vi "Live.GetChannelInfo.vi"(8 "error in (no error)":errorcluster, 10 "Item URL":string, 11 "OPC UA client refnum in":refnum<k21>) -> (0 "error out":errorcluster, 1 "Setings":T1={"Settings"={"name"="", "node type"=enum."Other", "DataType"=1, "access"=enum."Null", "description"=""}, "Array Size"=0} {"Settings"."DataType" items=["Boolean"=1, "SByte"=2, "Byte"=3, "Int16"=4, "UInt16"=5, "Int32"=6, "UInt32"=7, "Int64"=8, "UInt64"=9, "Float"=10, "Double"=11, "String"=12, "DateTime"=13, "ByteString"=15, "Array of Boolean"=101, "Array of SByte"=102, "Array of Byte"=103, "Array of Int16"=104, "Array of UInt16"=105, "Array of Int32"=106, "Array of UInt32"=107, "Array of Int64"=108, "Array of UInt64"=109, "Array of Float"=110, "Array of Double"=111, "Array of String"=112, "Array of DateTime"=113, "Array of ByteString"=115]}, 2 "Item URL out":string, 3 "OPC UA client refnum out":refnum<k21>, 4 "Use":bool)   [LabVIEW 2013, in "OPC UA Client System Explorer.lvlib"]
uses:
  OPC UA Client System Explorer.lvlib
  Types/Tag.Settings
  <vilib>/OPCUA/client/Read ByteString.vi
  <vilib>/OPCUA/client/Read Double Array.vi
  <vilib>/OPCUA/client/Read Float Array.vi
  <vilib>/OPCUA/client/Read UInt32 Array.vi
  <vilib>/OPCUA/client/Read Int32 Array.vi
  <vilib>/OPCUA/client/Read UInt16 Array.vi
  <vilib>/OPCUA/client/Read Int16 Array.vi
  <vilib>/OPCUA/client/Read Byte Array.vi
  <vilib>/OPCUA/client/Read SByte Array.vi
  <vilib>/OPCUA/client/Read Bool Array.vi
  <vilib>/OPCUA/client/Read UInt64 Array.vi
  <vilib>/OPCUA/client/Read Int64 Array.vi
  <vilib>/OPCUA/client/Read DateTime Array.vi
  Engine/OPC UA Client Engine.lvlib
  <vilib>/OPCUA/NI OPC UA Client.lvlib
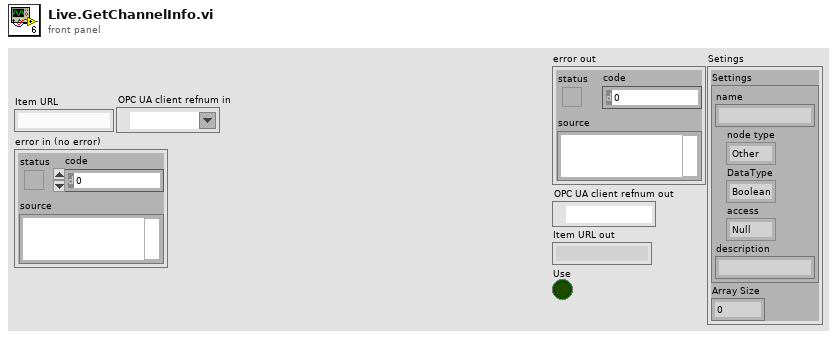
[diagram p1: front panel]
types:
  T1 = typedef "OPC UA Client Engine.lvlib/Tag.Settings" = cluster{"Settings":cluster{"name":string, "node type":enum32{"Other", "Folder", "Item/Property"}, "DataType":u32, "access":enum16{"Null", "Read", "Write", "Read&Write"}, "description":string}, "Array Size":i32}
  T2 = cluster{"name":string, "node type":enum32{"Other", "Folder", "Item/Property"}, "DataType":u32, "access":enum16{"Null", "Read", "Write", "Read&Write"}, "description":string}
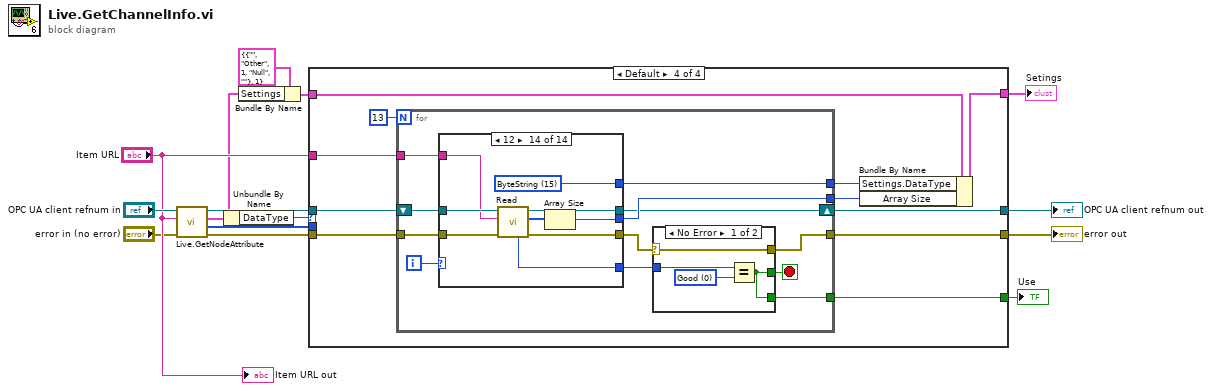
[diagram p0: block diagram]
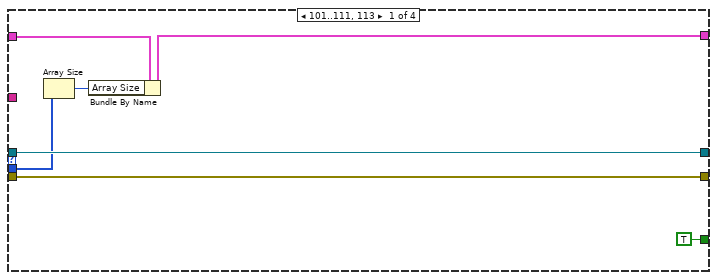
[diagram p2: hidden frame]
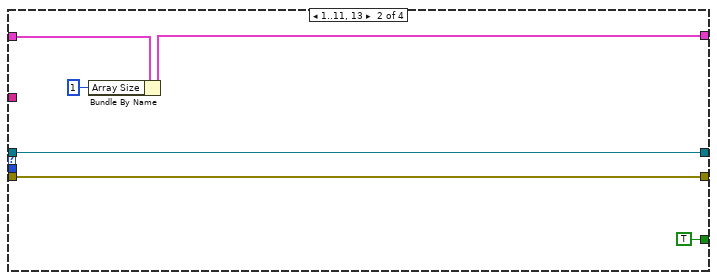
[diagram p3: hidden frame]
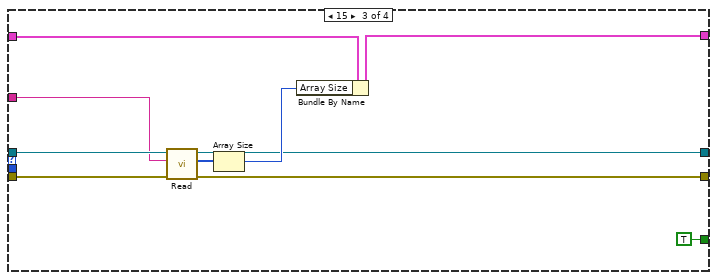
[diagram p4: hidden frame]
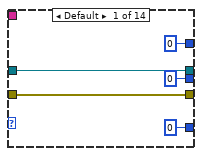
[diagram p5: hidden frame]
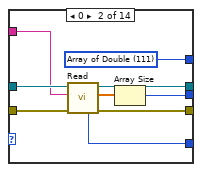
[diagram p6: hidden frame]
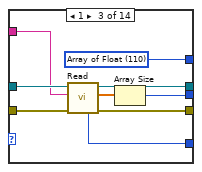
[diagram p7: hidden frame]
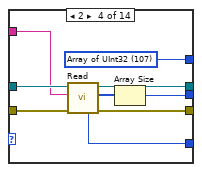
[diagram p8: hidden frame]
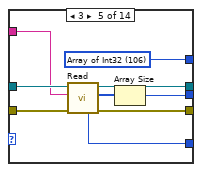
[diagram p9: hidden frame]
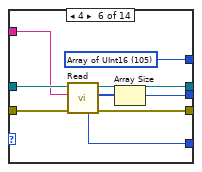
[diagram p10: hidden frame]
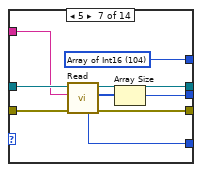
[diagram p11: hidden frame]
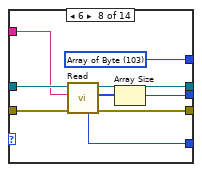
[diagram p12: hidden frame]
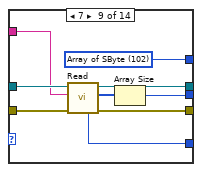
[diagram p13: hidden frame]
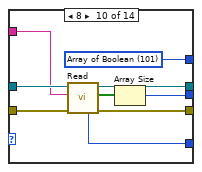
[diagram p14: hidden frame]
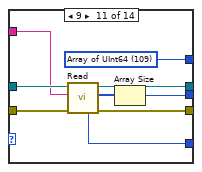
[diagram p15: hidden frame]
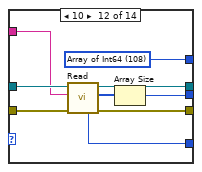
[diagram p16: hidden frame]
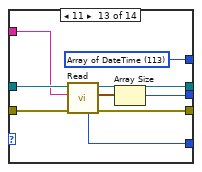
[diagram p17: hidden frame]
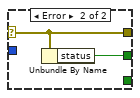
[diagram p18: hidden frame]
diagram:
  n1 = call "Live.GetNodeAttribute.vi"("error in (no error)"="error in (no error)", "node path"="Item URL", "OPC UA client refnum in"="OPC UA client refnum in") -> ("error out"=w6:errorcluster, "status"=w3:u32[], "node attribute"=w4:T2, "OPC UA client refnum out"=w5:refnum<k21>)  [unwired: 5 in]
  n2 = Unbundle By Name(w4) -> ("DataType"=w11:u32)
  n3 = Bundle By Name(cluster=T1 {"Settings"={"name"="", "node type"=enum."Other", "DataType"=1, "access"=enum."Null", "description"=""}, "Array Size"=1}, "Settings"=w4) -> (w10:T1)
  n4 = case shown="Default" w11 {
    tunnel: [w18 w24 w28 w40] -> w14
    tunnel: [w19 w25 w29 w39] -> w13
    tunnel: w6 -> [w18 w24 w33 w45]
    tunnel: w5 -> [w19 w25 w32 w43]
    tunnel: "Item URL" -> [_ _ w31 w44]
    tunnel: w10 -> [w21 w27 w37 w48]
    tunnel: [w20 w26 w36 w47] -> w2
    tunnel: w3 -> [w17 _ _ _]
    tunnel: [TRUE ("status") TRUE ("status") TRUE ("status") w38] -> w1
    frame 101..111, 113 {
      n5 = Array Size(array=w17) -> (size(s)=w16:i32)
      n6 = Bundle By Name(cluster=w21, "Array Size"=w16) -> (w20:T1)
    }
    frame 1..11, 13 {
      n7 = Bundle By Name(cluster=w27, "Array Size"=1) -> (w26:T1)
    }
    frame 15 {
      n8 = call-poly <vilib>:"Read.vi"("error in (no error)"=w33, "node path"=w31, "OPC UA client refnum in"=w32) -> ("error out"=w28:errorcluster, "value"=w34:u8[], "OPC UA client refnum out"=w29:refnum<k21>)  [unwired: 4 in, 2 out]
      n9 = Array Size(array=w34) -> (size(s)=w30:i32)
      n10 = Bundle By Name(cluster=w37, "Array Size"=w30) -> (w36:T1)
    }
    frame Default {
      n11 = for {
        N: 13 -> [_]
        tunnel: w45 -> [w60]
        tunnel: w44 -> [w58]
        tunnel: [w55] -> w40
        tunnel: [w53] -> w41
        tunnel: [w52] -> w42
        shift-right: [w51] -> w39
        shift-left: w43 -> [w59]
        tunnel: [w49] -> w38
        i -> [w54]
        stop <- w50 stop-if-true
        n12 = case shown="12" w54 {
          tunnel: w60 -> [w63 w74 w83 w92 w101 w110 w119 w128 w137 w146 w155 w164 w173 w182]
          tunnel: w59 -> [w61 w73 w82 w91 w100 w109 w118 w127 w136 w145 w154 w163 w172 w181]
          tunnel: w58 -> [_ w72 w81 w90 w99 w108 w117 w126 w135 w144 w153 w162 w171 w180]
          tunnel: [w63 w71 w80 w89 w98 w107 w116 w125 w134 w143 w152 w161 w170 w179] -> w57
          tunnel: [u32 0 ("status") w70 w79 w88 w97 w106 w115 w124 w133 w142 w151 w160 w169 w178] -> w56
          tunnel: [u32 0 ("DataType") w68 w77 w86 w95 w104 w113 w122 w131 w140 w149 w158 w167 w176] -> w52
          tunnel: [0 w67 w76 w85 w94 w103 w112 w121 w130 w139 w148 w157 w166 w175] -> w53
          tunnel: [w61 w66 w75 w84 w93 w102 w111 w120 w129 w138 w147 w156 w165 w174] -> w51
          frame Default {
          }
          frame 0 {
            w68 = u32 111 items=["Boolean"=1, "SByte"=2, "Byte"=3, "Int16"=4, "UInt16"=5, "Int32"=6, "UInt32"=7, "Int64"=8, "UInt64"=9, "Float"=10, "Double"=11, "String"=12, "DateTime"=13, "ByteString"=15, "Array of Boolean"=101, "Array of SByte"=102, "Array of Byte"=103, "Array of Int16"=104, "Array of UInt16"=105, "Array of Int32"=106, "Array of UInt32"=107, "Array of Int64"=108, "Array of UInt64"=109, "Array of Float"=110, "Array of Double"=111, "Array of String"=112, "Array of DateTime"=113, "Array of ByteString"=115] ("DataType")
            n13 = call-poly <vilib>:"Read.vi"("error in (no error)"=w74, "node path"=w72, "OPC UA client refnum in"=w73) -> ("error out"=w71:errorcluster, "value"=w69:dbl[], "OPC UA client refnum out"=w66:refnum<k21>, "status"=w70:u32)  [unwired: 4 in, 1 out]
            n14 = Array Size(array=w69) -> (size(s)=w67:i32)
          }
          frame 1 {
            w77 = u32 110 items=["Boolean"=1, "SByte"=2, "Byte"=3, "Int16"=4, "UInt16"=5, "Int32"=6, "UInt32"=7, "Int64"=8, "UInt64"=9, "Float"=10, "Double"=11, "String"=12, "DateTime"=13, "ByteString"=15, "Array of Boolean"=101, "Array of SByte"=102, "Array of Byte"=103, "Array of Int16"=104, "Array of UInt16"=105, "Array of Int32"=106, "Array of UInt32"=107, "Array of Int64"=108, "Array of UInt64"=109, "Array of Float"=110, "Array of Double"=111, "Array of String"=112, "Array of DateTime"=113, "Array of ByteString"=115] ("DataType")
            n15 = call-poly <vilib>:"Read.vi"("error in (no error)"=w83, "node path"=w81, "OPC UA client refnum in"=w82) -> ("error out"=w80:errorcluster, "value"=w78:sgl[], "OPC UA client refnum out"=w75:refnum<k21>, "status"=w79:u32)  [unwired: 4 in, 1 out]
            n16 = Array Size(array=w78) -> (size(s)=w76:i32)
          }
          frame 2 {
            w86 = u32 107 items=["Boolean"=1, "SByte"=2, "Byte"=3, "Int16"=4, "UInt16"=5, "Int32"=6, "UInt32"=7, "Int64"=8, "UInt64"=9, "Float"=10, "Double"=11, "String"=12, "DateTime"=13, "ByteString"=15, "Array of Boolean"=101, "Array of SByte"=102, "Array of Byte"=103, "Array of Int16"=104, "Array of UInt16"=105, "Array of Int32"=106, "Array of UInt32"=107, "Array of Int64"=108, "Array of UInt64"=109, "Array of Float"=110, "Array of Double"=111, "Array of String"=112, "Array of DateTime"=113, "Array of ByteString"=115] ("DataType")
            n17 = call-poly <vilib>:"Read.vi"("error in (no error)"=w92, "node path"=w90, "OPC UA client refnum in"=w91) -> ("error out"=w89:errorcluster, "value"=w87:u32[], "OPC UA client refnum out"=w84:refnum<k21>, "status"=w88:u32)  [unwired: 4 in, 1 out]
            n18 = Array Size(array=w87) -> (size(s)=w85:i32)
          }
          frame 3 {
            w95 = u32 106 items=["Boolean"=1, "SByte"=2, "Byte"=3, "Int16"=4, "UInt16"=5, "Int32"=6, "UInt32"=7, "Int64"=8, "UInt64"=9, "Float"=10, "Double"=11, "String"=12, "DateTime"=13, "ByteString"=15, "Array of Boolean"=101, "Array of SByte"=102, "Array of Byte"=103, "Array of Int16"=104, "Array of UInt16"=105, "Array of Int32"=106, "Array of UInt32"=107, "Array of Int64"=108, "Array of UInt64"=109, "Array of Float"=110, "Array of Double"=111, "Array of String"=112, "Array of DateTime"=113, "Array of ByteString"=115] ("DataType")
            n19 = call-poly <vilib>:"Read.vi"("error in (no error)"=w101, "node path"=w99, "OPC UA client refnum in"=w100) -> ("error out"=w98:errorcluster, "value"=w96:i32[], "OPC UA client refnum out"=w93:refnum<k21>, "status"=w97:u32)  [unwired: 4 in, 1 out]
            n20 = Array Size(array=w96) -> (size(s)=w94:i32)
          }
          frame 4 {
            w104 = u32 105 items=["Boolean"=1, "SByte"=2, "Byte"=3, "Int16"=4, "UInt16"=5, "Int32"=6, "UInt32"=7, "Int64"=8, "UInt64"=9, "Float"=10, "Double"=11, "String"=12, "DateTime"=13, "ByteString"=15, "Array of Boolean"=101, "Array of SByte"=102, "Array of Byte"=103, "Array of Int16"=104, "Array of UInt16"=105, "Array of Int32"=106, "Array of UInt32"=107, "Array of Int64"=108, "Array of UInt64"=109, "Array of Float"=110, "Array of Double"=111, "Array of String"=112, "Array of DateTime"=113, "Array of ByteString"=115] ("DataType")
            n21 = call-poly <vilib>:"Read.vi"("error in (no error)"=w110, "node path"=w108, "OPC UA client refnum in"=w109) -> ("error out"=w107:errorcluster, "value"=w105:u16[], "OPC UA client refnum out"=w102:refnum<k21>, "status"=w106:u32)  [unwired: 4 in, 1 out]
            n22 = Array Size(array=w105) -> (size(s)=w103:i32)
          }
          frame 5 {
            w113 = u32 104 items=["Boolean"=1, "SByte"=2, "Byte"=3, "Int16"=4, "UInt16"=5, "Int32"=6, "UInt32"=7, "Int64"=8, "UInt64"=9, "Float"=10, "Double"=11, "String"=12, "DateTime"=13, "ByteString"=15, "Array of Boolean"=101, "Array of SByte"=102, "Array of Byte"=103, "Array of Int16"=104, "Array of UInt16"=105, "Array of Int32"=106, "Array of UInt32"=107, "Array of Int64"=108, "Array of UInt64"=109, "Array of Float"=110, "Array of Double"=111, "Array of String"=112, "Array of DateTime"=113, "Array of ByteString"=115] ("DataType")
            n23 = call-poly <vilib>:"Read.vi"("error in (no error)"=w119, "node path"=w117, "OPC UA client refnum in"=w118) -> ("error out"=w116:errorcluster, "value"=w114:i16[], "OPC UA client refnum out"=w111:refnum<k21>, "status"=w115:u32)  [unwired: 4 in, 1 out]
            n24 = Array Size(array=w114) -> (size(s)=w112:i32)
          }
          frame 6 {
            w122 = u32 103 items=["Boolean"=1, "SByte"=2, "Byte"=3, "Int16"=4, "UInt16"=5, "Int32"=6, "UInt32"=7, "Int64"=8, "UInt64"=9, "Float"=10, "Double"=11, "String"=12, "DateTime"=13, "ByteString"=15, "Array of Boolean"=101, "Array of SByte"=102, "Array of Byte"=103, "Array of Int16"=104, "Array of UInt16"=105, "Array of Int32"=106, "Array of UInt32"=107, "Array of Int64"=108, "Array of UInt64"=109, "Array of Float"=110, "Array of Double"=111, "Array of String"=112, "Array of DateTime"=113, "Array of ByteString"=115] ("DataType")
            n25 = call-poly <vilib>:"Read.vi"("error in (no error)"=w128, "node path"=w126, "OPC UA client refnum in"=w127) -> ("error out"=w125:errorcluster, "value"=w123:u8[], "OPC UA client refnum out"=w120:refnum<k21>, "status"=w124:u32)  [unwired: 4 in, 1 out]
            n26 = Array Size(array=w123) -> (size(s)=w121:i32)
          }
          frame 7 {
            w131 = u32 102 items=["Boolean"=1, "SByte"=2, "Byte"=3, "Int16"=4, "UInt16"=5, "Int32"=6, "UInt32"=7, "Int64"=8, "UInt64"=9, "Float"=10, "Double"=11, "String"=12, "DateTime"=13, "ByteString"=15, "Array of Boolean"=101, "Array of SByte"=102, "Array of Byte"=103, "Array of Int16"=104, "Array of UInt16"=105, "Array of Int32"=106, "Array of UInt32"=107, "Array of Int64"=108, "Array of UInt64"=109, "Array of Float"=110, "Array of Double"=111, "Array of String"=112, "Array of DateTime"=113, "Array of ByteString"=115] ("DataType")
            n27 = call-poly <vilib>:"Read.vi"("error in (no error)"=w137, "node path"=w135, "OPC UA client refnum in"=w136) -> ("error out"=w134:errorcluster, "value"=w132:i8[], "OPC UA client refnum out"=w129:refnum<k21>, "status"=w133:u32)  [unwired: 4 in, 1 out]
            n28 = Array Size(array=w132) -> (size(s)=w130:i32)
          }
          frame 8 {
            w140 = u32 101 items=["Boolean"=1, "SByte"=2, "Byte"=3, "Int16"=4, "UInt16"=5, "Int32"=6, "UInt32"=7, "Int64"=8, "UInt64"=9, "Float"=10, "Double"=11, "String"=12, "DateTime"=13, "ByteString"=15, "Array of Boolean"=101, "Array of SByte"=102, "Array of Byte"=103, "Array of Int16"=104, "Array of UInt16"=105, "Array of Int32"=106, "Array of UInt32"=107, "Array of Int64"=108, "Array of UInt64"=109, "Array of Float"=110, "Array of Double"=111, "Array of String"=112, "Array of DateTime"=113, "Array of ByteString"=115] ("DataType")
            n29 = call-poly <vilib>:"Read.vi"("error in (no error)"=w146, "node path"=w144, "OPC UA client refnum in"=w145) -> ("error out"=w143:errorcluster, "value"=w141:bool[], "OPC UA client refnum out"=w138:refnum<k21>, "status"=w142:u32)  [unwired: 4 in, 1 out]
            n30 = Array Size(array=w141) -> (size(s)=w139:i32)
          }
          frame 9 {
            w149 = u32 109 items=["Boolean"=1, "SByte"=2, "Byte"=3, "Int16"=4, "UInt16"=5, "Int32"=6, "UInt32"=7, "Int64"=8, "UInt64"=9, "Float"=10, "Double"=11, "String"=12, "DateTime"=13, "ByteString"=15, "Array of Boolean"=101, "Array of SByte"=102, "Array of Byte"=103, "Array of Int16"=104, "Array of UInt16"=105, "Array of Int32"=106, "Array of UInt32"=107, "Array of Int64"=108, "Array of UInt64"=109, "Array of Float"=110, "Array of Double"=111, "Array of String"=112, "Array of DateTime"=113, "Array of ByteString"=115] ("DataType")
            n31 = call-poly <vilib>:"Read.vi"("error in (no error)"=w155, "node path"=w153, "OPC UA client refnum in"=w154) -> ("error out"=w152:errorcluster, "value"=w150:u64[], "OPC UA client refnum out"=w147:refnum<k21>, "status"=w151:u32)  [unwired: 4 in, 1 out]
            n32 = Array Size(array=w150) -> (size(s)=w148:i32)
          }
          frame 10 {
            w158 = u32 108 items=["Boolean"=1, "SByte"=2, "Byte"=3, "Int16"=4, "UInt16"=5, "Int32"=6, "UInt32"=7, "Int64"=8, "UInt64"=9, "Float"=10, "Double"=11, "String"=12, "DateTime"=13, "ByteString"=15, "Array of Boolean"=101, "Array of SByte"=102, "Array of Byte"=103, "Array of Int16"=104, "Array of UInt16"=105, "Array of Int32"=106, "Array of UInt32"=107, "Array of Int64"=108, "Array of UInt64"=109, "Array of Float"=110, "Array of Double"=111, "Array of String"=112, "Array of DateTime"=113, "Array of ByteString"=115] ("DataType")
            n33 = call-poly <vilib>:"Read.vi"("error in (no error)"=w164, "node path"=w162, "OPC UA client refnum in"=w163) -> ("error out"=w161:errorcluster, "value"=w159:i64[], "OPC UA client refnum out"=w156:refnum<k21>, "status"=w160:u32)  [unwired: 4 in, 1 out]
            n34 = Array Size(array=w159) -> (size(s)=w157:i32)
          }
          frame 11 {
            w167 = u32 113 items=["Boolean"=1, "SByte"=2, "Byte"=3, "Int16"=4, "UInt16"=5, "Int32"=6, "UInt32"=7, "Int64"=8, "UInt64"=9, "Float"=10, "Double"=11, "String"=12, "DateTime"=13, "ByteString"=15, "Array of Boolean"=101, "Array of SByte"=102, "Array of Byte"=103, "Array of Int16"=104, "Array of UInt16"=105, "Array of Int32"=106, "Array of UInt32"=107, "Array of Int64"=108, "Array of UInt64"=109, "Array of Float"=110, "Array of Double"=111, "Array of String"=112, "Array of DateTime"=113, "Array of ByteString"=115] ("DataType")
            n35 = call-poly <vilib>:"Read.vi"("error in (no error)"=w173, "node path"=w171, "OPC UA client refnum in"=w172) -> ("error out"=w170:errorcluster, "value"=w168:timestamp[], "OPC UA client refnum out"=w165:refnum<k21>, "status"=w169:u32)  [unwired: 4 in, 1 out]
            n36 = Array Size(array=w168) -> (size(s)=w166:i32)
          }
          frame 12 {
            w176 = u32 15 items=["Boolean"=1, "SByte"=2, "Byte"=3, "Int16"=4, "UInt16"=5, "Int32"=6, "UInt32"=7, "Int64"=8, "UInt64"=9, "Float"=10, "Double"=11, "String"=12, "DateTime"=13, "ByteString"=15, "Array of Boolean"=101, "Array of SByte"=102, "Array of Byte"=103, "Array of Int16"=104, "Array of UInt16"=105, "Array of Int32"=106, "Array of UInt32"=107, "Array of Int64"=108, "Array of UInt64"=109, "Array of Float"=110, "Array of Double"=111, "Array of String"=112, "Array of DateTime"=113, "Array of ByteString"=115] ("DataType")
            n37 = call-poly <vilib>:"Read.vi"("error in (no error)"=w182, "node path"=w180, "OPC UA client refnum in"=w181) -> ("error out"=w179:errorcluster, "value"=w177:u8[], "OPC UA client refnum out"=w174:refnum<k21>, "status"=w178:u32)  [unwired: 4 in, 1 out]
            n38 = Array Size(array=w177) -> (size(s)=w175:i32)
          }
        }
        n39 = case shown="No Error" w57 {
          selector: w57 -> [w184 w187]
          tunnel: w56 -> [w186 _]
          tunnel: [w183 w188] -> w50
          tunnel: [w184 w187] -> w55
          tunnel: [w183 _] -> w49
          frame No Error {
            w185 = u32 0 items=["Good"=0, "Bad_AttributeIdInvalid"=2153906176, "Bad_BrowseDirectionInvalid"=2152529920, "Bad_BrowseNameInvalid"=2153775104, "Bad_ContentFilterInvalid"=2152202240, "Bad_ContinuationPointInvalid"=2152333312, "Bad_DataEncodingInvalid"=2151153664, "Bad_DataEncodingUnsupported"=2151219200, "Bad_EventFilterInvalid"=2152136704, "Bad_FilterNotAllowed"=2152005632, "Bad_FilterOperandInvalid"=2160132096, "Bad_HistoryOperationInvalid"=2154889216, "Bad_HistoryOperationUnsupported"=2154954752, "Bad_IndexRangeInvalid"=2151022592, "Bad_IndexRangeNoData"=2151088128, "Bad_MonitoredItemFilterInvalid"=2151874560, "Bad_MonitoredItemFilterUnsupported"=2151940096, "Bad_MonitoredItemIdInvalid"=2151809024, "Bad_MonitoringModeInvalid"=2151743488, "Bad_NoCommunication"=2150694912, "Bad_NoContinuationPoints"=2152398848, "Bad_NodeClassInvalid"=2153709568, "Bad_NodeIdInvalid"=2150825984, "Bad_NodeIdUnknown"=2150891520, "Bad_NoDeleteRights"=2154364928, "Bad_NodeNotInView"=2152595456, "Bad_NotFound"=2151546880, "Bad_NotImplemented"=2151677952, "Bad_NotReadable"=2151284736, "Bad_NotSupported"=2151481344, "Bad_NotWritable"=2151350272, "Bad_ObjectDeleted"=2151612416, "Bad_OutOfRange"=2151415808, "Bad_ReferenceTypeIdInvalid"=2152464384, "Bad_SourceNodeIdInvalid"=2154037248, "Bad_StructureMissing"=2152071168, "Bad_TargetNodeIdInvalid"=2154102784, "Bad_TypeDefinitionInvalid"=2153971712, "Bad_TypeMismatch"=2155085824, "Bad_WaitingForInitialData"=2150760448] ("status")
            n40 = Equal?(x=w186, y=w185) -> (x = y?=w183:bool)
          }
          frame Error {
            n41 = Unbundle By Name(w187) -> ("status"=w188:bool)
          }
        }
      }
      n42 = Bundle By Name(cluster=w48, "Settings.DataType"=w42, "Array Size"=w41) -> (w47:T1)
    }
  }
  "error out" <- w14
  "OPC UA client refnum out" <- w13
  "Setings" <- w2
  "Use" <- w1
  "Item URL out" <- "Item URL"
